vi "SetSourceDelay.vi"(7 "SMU":T2, 8 "Error In":errorcluster, 9 "User Value (sec)":dbl, 10 "Source Delay Type":T1, 11 "Keithley 2602 In":refnum<visa-resource-name>) -> (0 "Error Out":errorcluster, 3 "Keithley 2602 Out":refnum<visa-resource-name>)   [LabVIEW 2012, in "Keithley-2602.lvlib"]
uses:
  Keithley-2602.lvlib
  Controls/SMU.ctl
  Controls/SourceDelayType.ctl
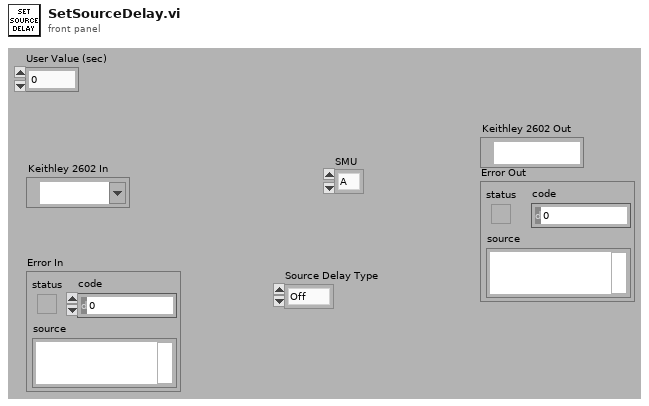
[diagram p1: front panel]
types:
  T1 = typedef "Keithley-2602.lvlib/SourceDelayType.ctl" = enum16{"Off", "Auto", "User"}
  T2 = typedef "Keithley-2602.lvlib/SMU.ctl" = enum16{"A", "B"}
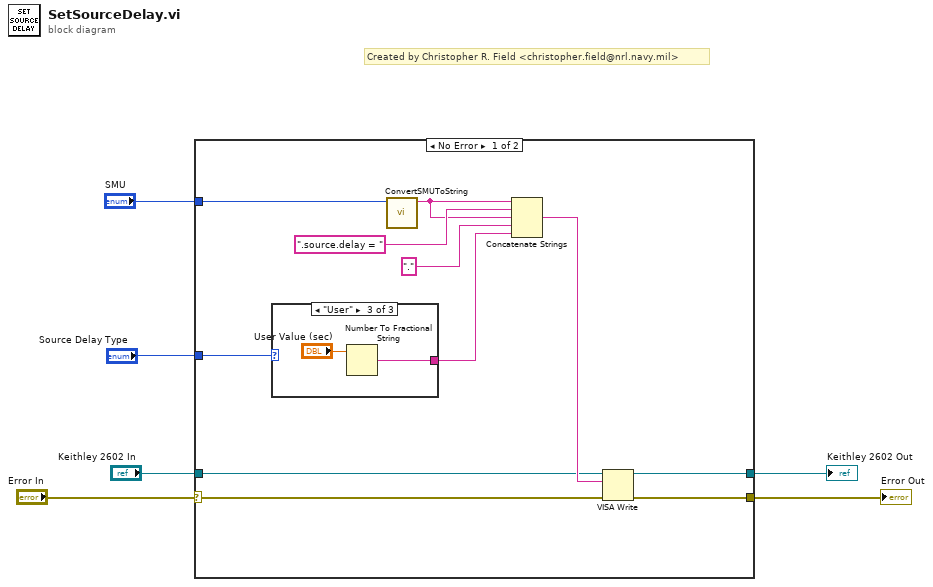
[diagram p0: block diagram]
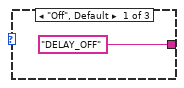
[diagram p2: hidden frame]
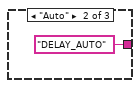
[diagram p3: hidden frame]
diagram:
  # "Created by Christopher R. Field <christopher.field@nrl.navy.mil>"
  n1 = case shown="No Error" "Error In" {
    selector: "Error In" -> [w7 w22]
    tunnel: "Keithley 2602 In" -> [w12 w23]
    tunnel: [w11 w23] -> w5
    tunnel: [w10 w22] -> w4
    tunnel: "Source Delay Type" -> [w9 _]
    tunnel: "SMU" -> [w8 _]
    frame No Error {
      n2 = case shown="\"User\"" w9 {
        tunnel: ["DELAY_OFF" "DELAY_AUTO" w21] -> w14
        frame "Off", Default {
        }
        frame "Auto" {
        }
        frame "User" {
          n3 = Number To Fractional String(number="User Value (sec)") -> (F-format string=w21:string)  [unwired: 3 in]
        }
      }
      n4 = call "ConvertSMUToString.vi"("SMU"=w8) -> ("Channel"=w16:string)  [unwired: 10 in]
      n5 = Concatenate Strings(w16, ".source.delay = ", w16, "." ("string"), w14) -> (w13:string)
      n6 = VISA Write(VISA resource name=w12, write buffer=w13, error in (no error)=w7) -> (VISA resource name out=w11:refnum<visa-resource-name>, error out=w10:errorcluster)  [unwired: 1 out]
    }
    frame Error {
    }
  }
  "Keithley 2602 Out" <- w5
  "Error Out" <- w4
